vi "CommonVIs ClassItemStringParser.vi"(0 "ClassItemNameIn":string) -> (14 "Class":string, 15 "Name":string)   [LabVIEW 2014]
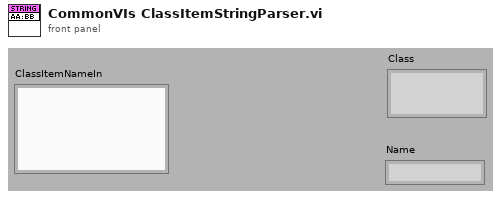
[diagram p1: front panel]
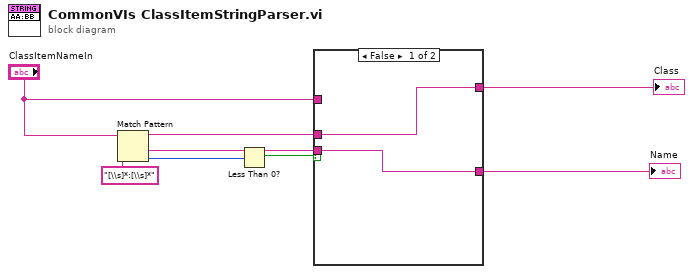
[diagram p0: block diagram]
diagram:
  n1 = Match Pattern(string="ClassItemNameIn", regular expression="[\\s]*:[\\s]*") -> (before substring=w3:string, after substring=w1:string, offset past match=w7:i32)  [unwired: 2 out]
  n2 = Less Than 0?(x=w7) -> (x < 0?=w6:bool)
  n3 = case shown="False" w6 {
    tunnel: "ClassItemNameIn" -> [_ w11]
    tunnel: [w9 w11] -> w4
    tunnel: w3 -> [w10 _]
    tunnel: [w10 _] -> w2
    tunnel: w1 -> [w9 _]
    frame False {
    }
    frame True {
    }
  }
  "Class" <- w2
  "Name" <- w4
